vi "FTW-Time-Uptime.vi"(11 "error in":errorcluster) -> (4 "Current Uptime":dbl format="%.3fmsec\n%<%D:%H:%M:%S%3u>t", 15 "error out":errorcluster)   [LabVIEW 2012]
panel:
  # "Inputs"
  # "Outputs"
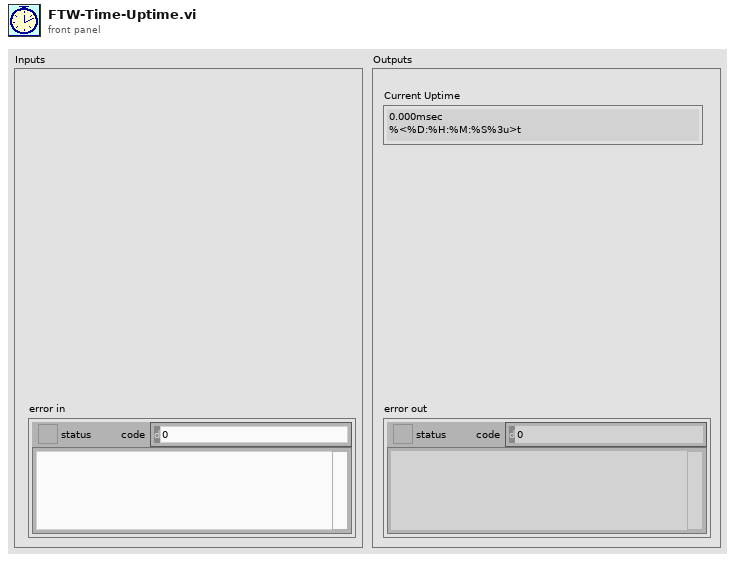
[diagram p1: front panel]
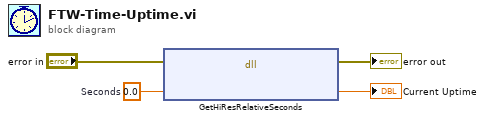
[diagram p0: block diagram]
diagram:
  w4 = 0.0  # Seconds
  n1 = dll-call lib="LabVIEW" fn="GetHiResRelativeSeconds"(error in="error in", "Seconds"=w4) -> (error out=→"error out":errorcluster, "Seconds"=→"Current Uptime":dbl)  [unwired: 3 in, 1 out]
